vi "Get Full Terminal Name.vi"(8 "error in":errorcluster, 10 "Local Terminal Name":string, 11 "task/channels in":refnum<k21>) -> (0 "error out":errorcluster, 2 "Terminal Name with Device Prefix":tag, 3 "task out":refnum<k21>)   [LabVIEW 2022 SP3]
doc: "This example takes in a DAQmx Task and a terminal and converts this to a terminal which includes the device prefix specified in the DAQmx Physical Channel Control.\n\nFor example: \nDAQmx Task/channels in=Dev1/ai1:2\nTerminal=ai/StartTrigger\nDevice+Terminal=/Dev1/ai/StartTrigger"
uses:
  <resource>/objmgr/daqmx.rc
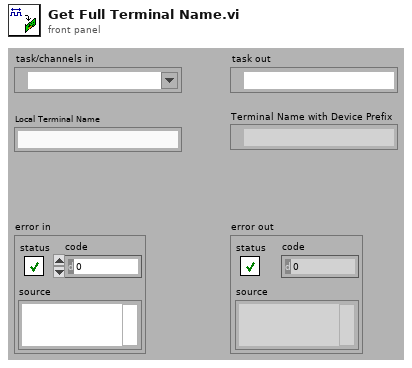
[diagram p1: front panel]
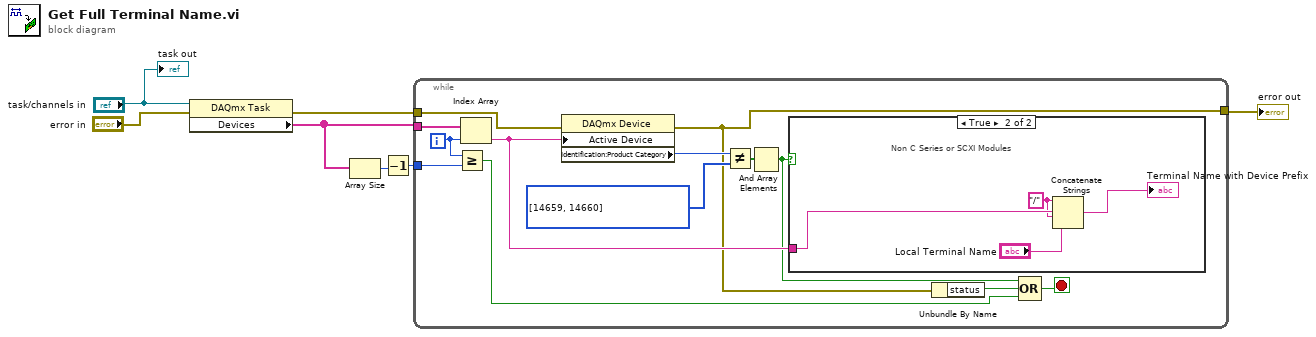
[diagram p0: block diagram]
diagram:
  n1 = property class="DAQmx Task"(reference="task/channels in", error in="error in") -> (error out=w5:errorcluster, "Devices"=w3:tag[])  [unwired: 1 out]
  n2 = Array Size(array=w3) -> (size(s)=w2:i32)
  n3 = Decrement(x=w2) -> (x-1=w1:i32)
  n4 = while {
    tunnel: w3 -> [w20]
    tunnel: w5 -> [w15]
    tunnel: [w14] -> w4
    tunnel: w1 -> [w12]
    i -> [w13]
    stop <- w8 stop-if-true
    w18 = i32[] [14659, 14660] items=["M Series DAQ"=14643, "E Series DAQ"=14642, "S Series DAQ"=14644, "B Series DAQ"=14662, "SC Series DAQ"=14645, "USB DAQ"=14646, "AO Series"=14647, "Digital I/O"=14648, "TIO Series"=14661, "Dynamic Signal Acquisition"=14649, "Switches"=14650, "C Series Chassis"=14658, "C Series Module"=14659, "SCXI Module"=14660, "Unknown"=12588]
    n5 = Greater Or Equal?(x=w13, y=w12) -> (x >= y?=w9:bool)
    n6 = Index Array(array=w20, index=w13) -> (element=w16:tag)
    n7 = property class="DAQmx Device"(error in=w15, "Active Device"=w16) -> (error out=w14:errorcluster, "Identification:Product Category"=w19:i32)  [unwired: 1 in, 1 out]
    n8 = Not Equal?(x=w19, y=w18) -> (x != y?=w17:bool[])
    n9 = And Array Elements(Boolean array=w17) -> (logical AND=w11:bool)
    n10 = case shown="True" w11 {
      tunnel: w16 -> [_ w24]
      frame False {
        # "Module Case do nothing"
      }
      frame True {
        w23 = "/" ("string")
        # "Non C Series or SCXI Modules"
        n11 = Concatenate Strings(w23, w24, w23, "Local Terminal Name") -> (→"Terminal Name with Device Prefix":string)
      }
    }
    n12 = Unbundle By Name(w14) -> ("status"=w10:bool)
    n13 = Compound Arithmetic op=OR(w11, w10, w9) -> (w8:bool)
  }
  "error out" <- w4
  "task out" <- "task/channels in"
